vi "Raman Spectrometer Controller GFV.vi"(0 "Data in":variant, 1 "SpectrometerEnum":T1=enum."MeasurementCompleted?", 3 "error in (no error)":errorcluster) -> (7 "Data Out":variant, 10 "error out":errorcluster)   [LabVIEW 2017]
doc: "Use this template to build a VI to use as a subVI."
uses:
  Spectrometer Utilities/SpectrometerControllerEnum.ctl
  Spectrometer Utilities/SpectrometerData.ctl
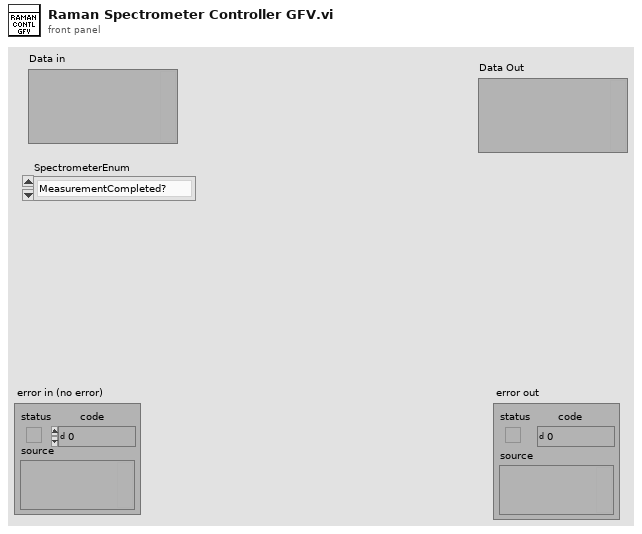
[diagram p1: front panel]
types:
  T1 = typedef "SpectrometerControllerEnum.ctl" = enum16{"Init!", "Start!", "Stop!", "Start New Measurement!", "MeasurementCompleted?", "Update Current Measurement Data", "Get Current Measurement Data!", "GetSpectrometerVIRef!"}
  T2 = typedef "SpectrometerData.ctl" = cluster{"Acquisition Time":dbl, "Range Begin":dbl, "Acquistion Time Unit":string, "Accumulations":i32, "Range End":dbl, "Range Unit":string, "Windows":i32, "Auto Focus":bool, "Auto Exposure":bool, "Spike Filter":string, "Delay Time":dbl, "Delay Time Unit":string, "Binning":i32, "Readout Mode":string, "DeNoise":bool, "ICS correction":bool, "Dark correction":bool, "Instrument Process":bool, "Instrument":string, "Detector":string, "Objective":string, "Grating":i32, "Grating Unit":string, "ND Filter":dbl, "ND Filter Unit":string, "Laser":dbl, "Laser Unit":string, "Slit":dbl, "Hole":dbl, "Acquired DateTime":string, "X axis":dbl[], "Y axis":dbl[]}
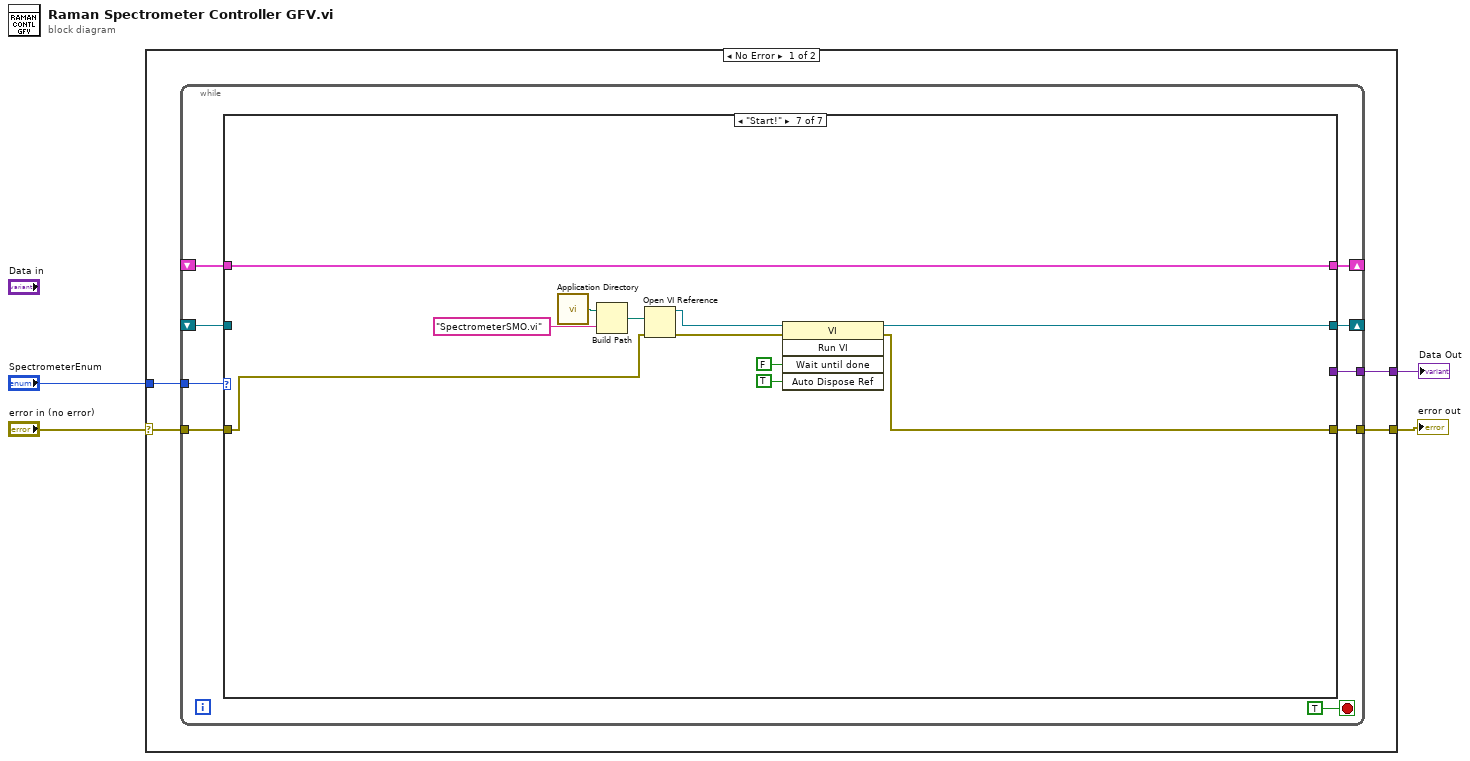
[diagram p0: block diagram]
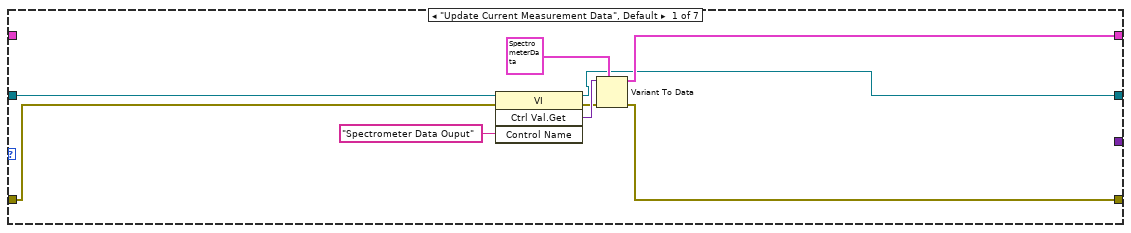
[diagram p2: hidden frame]
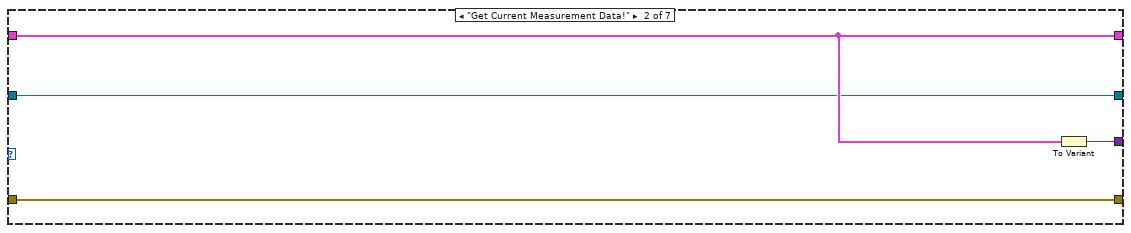
[diagram p3: hidden frame]
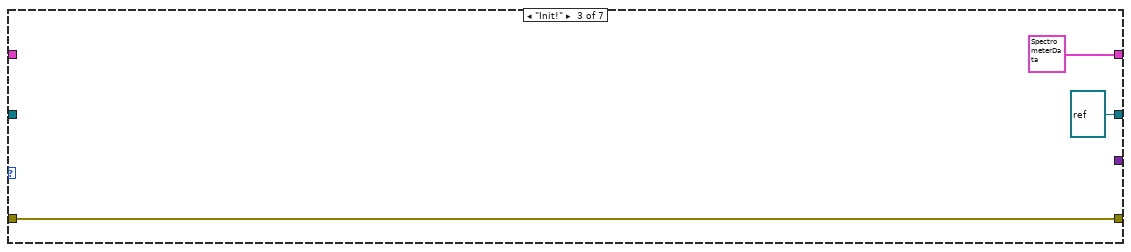
[diagram p4: hidden frame]
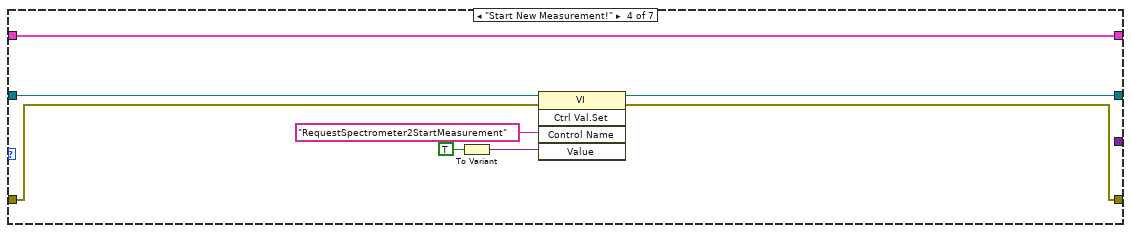
[diagram p5: hidden frame]
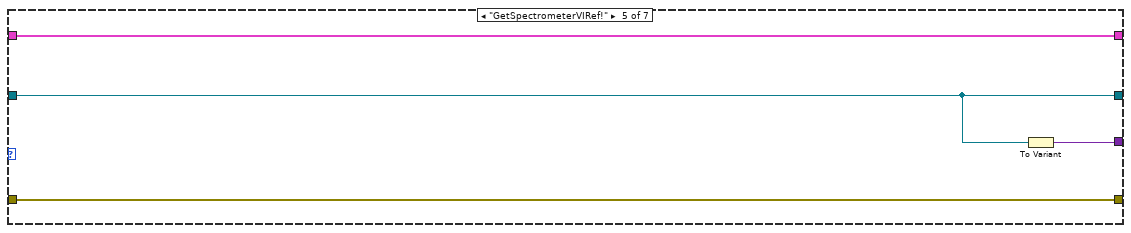
[diagram p6: hidden frame]
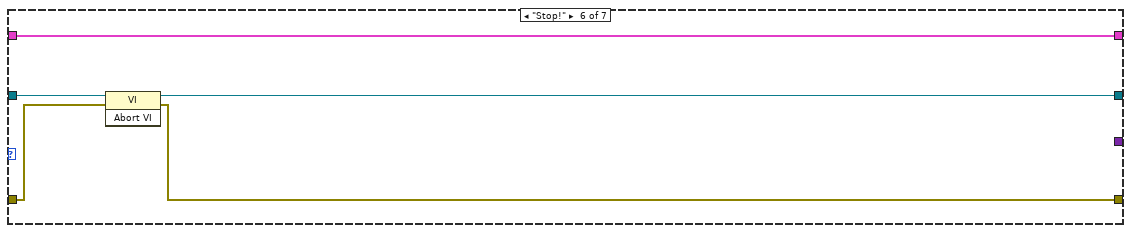
[diagram p7: hidden frame]
diagram:
  n1 = case shown="No Error" "error in (no error)" {
    selector: "error in (no error)" -> [w7 w62]
    tunnel: [w6 w62] -> w3
    tunnel: "SpectrometerEnum" -> [w8 _]
    tunnel: [w5 _] -> w1
    frame No Error {
      n2 = while {
        tunnel: w8 -> [w16]
        shift-right: [w15] -> _
        shift-left: _ -> [w14]
        shift-right: [w13] -> _
        shift-left: _ -> [w12]
        tunnel: w7 -> [w11]
        tunnel: [w10] -> w6
        tunnel: [w9] -> w5
        stop <- TRUE stop-if-true
        n3 = case shown="\"Start!\"" w16 {
          tunnel: [w21 w29 T2 {"Acquisition Time"=0.0, "Range Begin"=0.0, "Acquistion Time Unit"="", "Accumulations"=0, "Range End"=0.0, "Range Unit"="", "Windows"=0, "Auto Focus"=FALSE, "Auto Exposure"=FALSE, "Spike Filter"="", "Delay Time"=0.0, "Delay Time Unit"="", "Binning"=0, "Readout Mode"="", "DeNoise"=FALSE, "ICS correction"=FALSE, "Dark correction"=FALSE, "Instrument Process"=FALSE, "Instrument"="", "Detector"="", "Objective"="", "Grating"=0, "Grating Unit"="", "ND Filter"=0.0, "ND Filter Unit"="", "Laser"=0.0, "Laser Unit"="", "Slit"=0.0, "Hole"=0.0, "Acquired DateTime"="", "X axis"=[], "Y axis"=[]} ("Spectrometer Data") w36 w45 w46 w56] -> w15
          tunnel: w14 -> [_ w29 _ w36 w45 w46 w56]
          tunnel: [w18 w28 refnum<vi> refnum ("vi reference") w37 w44 w47 w55] -> w13
          tunnel: w12 -> [w22 w28 _ w38 w44 w50 _]
          tunnel: w11 -> [w20 w27 w31 w34 w42 w49 w54]
          tunnel: [w19 w27 w31 w35 w42 w48 w53] -> w10
          tunnel: [_ w30 _ _ w43 _ _] -> w9
          frame "Update Current Measurement Data", Default {
            n4 = invoke class="VI" method="Ctrl Val.Get"(reference=w22, error in=w20, "Control Name"="Spectrometer Data Ouput") -> (reference out=w18:refnum<vi>, error out=w25:errorcluster, "Get Control Value Variant"=w26:variant)  [unwired: 1 in, 1 out]
            n5 = Variant To Data(error in=w25, type=T2 {"Acquisition Time"=0.0, "Range Begin"=0.0, "Acquistion Time Unit"="", "Accumulations"=0, "Range End"=0.0, "Range Unit"="", "Windows"=0, "Auto Focus"=FALSE, "Auto Exposure"=FALSE, "Spike Filter"="", "Delay Time"=0.0, "Delay Time Unit"="", "Binning"=0, "Readout Mode"="", "DeNoise"=FALSE, "ICS correction"=FALSE, "Dark correction"=FALSE, "Instrument Process"=FALSE, "Instrument"="", "Detector"="", "Objective"="", "Grating"=0, "Grating Unit"="", "ND Filter"=0.0, "ND Filter Unit"="", "Laser"=0.0, "Laser Unit"="", "Slit"=0.0, "Hole"=0.0, "Acquired DateTime"="", "X axis"=[], "Y axis"=[]} ("Spectrometer Data"), Variant=w26) -> (data=w21:T2, error out=w19:errorcluster)
          }
          frame "Get Current Measurement Data!" {
            n6 = To Variant(anything=w29) -> (Variant=w30:variant)
          }
          frame "Init!" {
          }
          frame "Start New Measurement!" {
            n7 = To Variant(anything=TRUE) -> (Variant=w40:variant)
            n8 = invoke class="VI" method="Ctrl Val.Set"(reference=w38, error in=w34, "Control Name"="RequestSpectrometer2StartMeasurement", "Value"=w40) -> (reference out=w37:refnum<vi>, error out=w35:errorcluster)  [unwired: 1 in, 3 out]
          }
          frame "GetSpectrometerVIRef!" {
            n9 = To Variant(anything=w44) -> (Variant=w43:variant)
          }
          frame "Stop!" {
            n10 = invoke class="VI" method="Abort VI"(reference=w50, error in=w49) -> (reference out=w47:refnum<vi>, error out=w48:errorcluster)  [unwired: 1 in, 1 out]
          }
          frame "Start!" {
            n11 = call <vilib>:"Application Directory.vi"() -> ("Application Directory"=w59:path)
            n12 = Build Path(base path=w59, name or relative path="SpectrometerSMO.vi") -> (appended path=w57:path)
            n13 = Open VI Reference(vi path=w57, error in (no error)=w54) -> (vi reference=w51:refnum<vi>, error out=w52:errorcluster)  [unwired: 4 in]
            n14 = invoke class="VI" method="Run VI"(reference=w51, error in=w52, "Wait until done"=FALSE ("Wait Until Done"), "Auto Dispose Ref"=TRUE ("Auto Dispose Reference")) -> (reference out=w55:refnum<vi>, error out=w53:errorcluster)  [unwired: 1 in, 3 out]
          }
        }
      }
    }
    frame Error {
    }
  }
  "error out" <- w3
  "Data Out" <- w1
